vi "SensorIntensidad_Final.vi"() -> ()   [LabVIEW 2024]
uses:
  <vilib>/userDefined/High Color/IMAQdx.ctl
  <vilib>/vision/driver/IMAQdx.llb/IMAQdx Buffer Number Mode.ctl
  <vilib>/vision/driver/IMAQdx.llb/IMAQdx Acquisition Mode.ctl
  <vilib>/express/express shared/transition.llb/Dynamic To Waveform Array.vi
  <vilib>/express/express signal manip/GetorSetDDTAttributes/Set DDT Attributes/SetT0.vi
  <vilib>/express/express shared/transition.llb/Waveform Array To Dynamic.vi
  <vilib>/express/express signal manip/GetorSetDDTAttributes/Set DDT Attributes/Set DDT Properties.xnode
  <vilib>/vision/driver/NI_Vision_Acquisition_Software.lvlib
  <vilib>/vision/NI_Vision_Development_Module.lvlib
panel:
  out "XY Graph":cluster{"Run Time (ms)":u32, "IM":sgl}[](graph)
  out "IM":sgl
  out "Rec":T1 {"Rotation" format="%.2f"; "Left" scale=0.0..1024.0; "Right" scale=0.0..1024.0}
  in  "Buffer Mode":T2
  in  "Cancel Button":bool
  out "frame rate (fps)":u32
  out "Run Time (ms)":u32
  out "ms timer":u32
  in  "Session In":T3
  out "Image":T4(plugin-control)
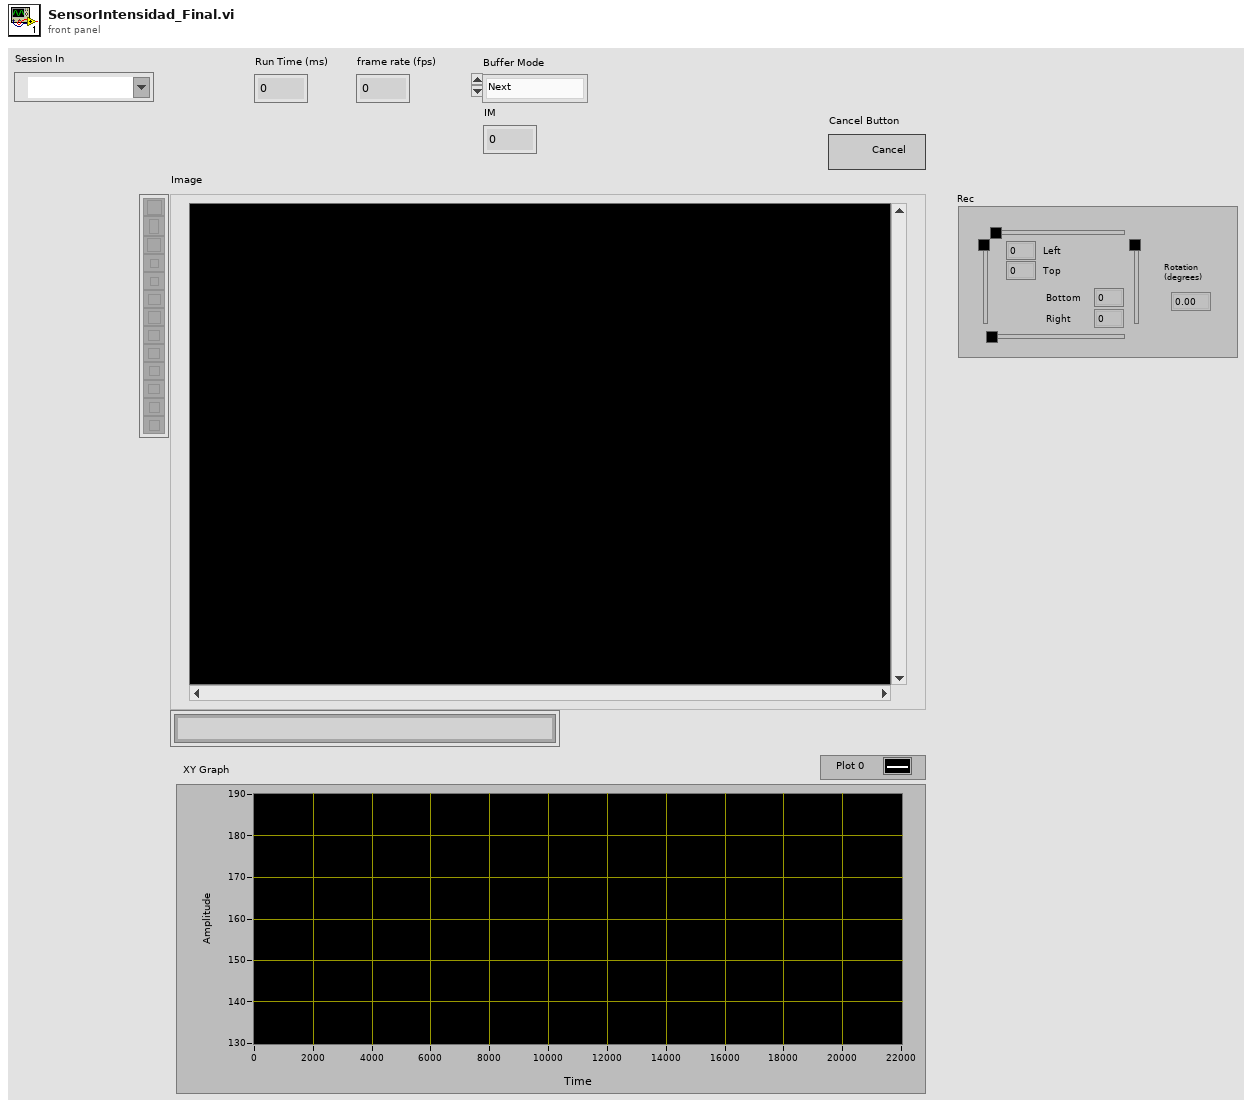
[diagram p1: front panel]
types:
  T1 = typedef "IMAQ Rectangle" = cluster{"Left":i32, "Top":i32, "Right":i32, "Bottom":i32, "Rotation":dbl}
  T2 = typedef "NI_Vision_Acquisition_Software.lvlib/IMAQdx Buffer Number Mode.ctl" = enum32{"Next", "Last", "Buffer Number", "Every", "Last New"}
  T3 = typedef "IMAQdx.ctl" = refnum<k21>
  T4 = typedef "IMAQ Image.ctl" = refnum<image>
  T5 = typedef "Image Type" = u32
  T6 = typedef "NI_Vision_Acquisition_Software.lvlib/IMAQdx Acquisition Mode.ctl" = enum32{"One Shot", "Continuous"}
  T7 = cluster{"Global Rectangle":i32[], "Contours":cluster{"Contour Type":u32, "ROI Type":u32, "Points":i32[]}[]}
  T8 = cluster{"Mean Intensity":sgl, "Standard  Deviation":sgl, "Minimum Intensity":sgl, "Maximum Intensity":sgl}
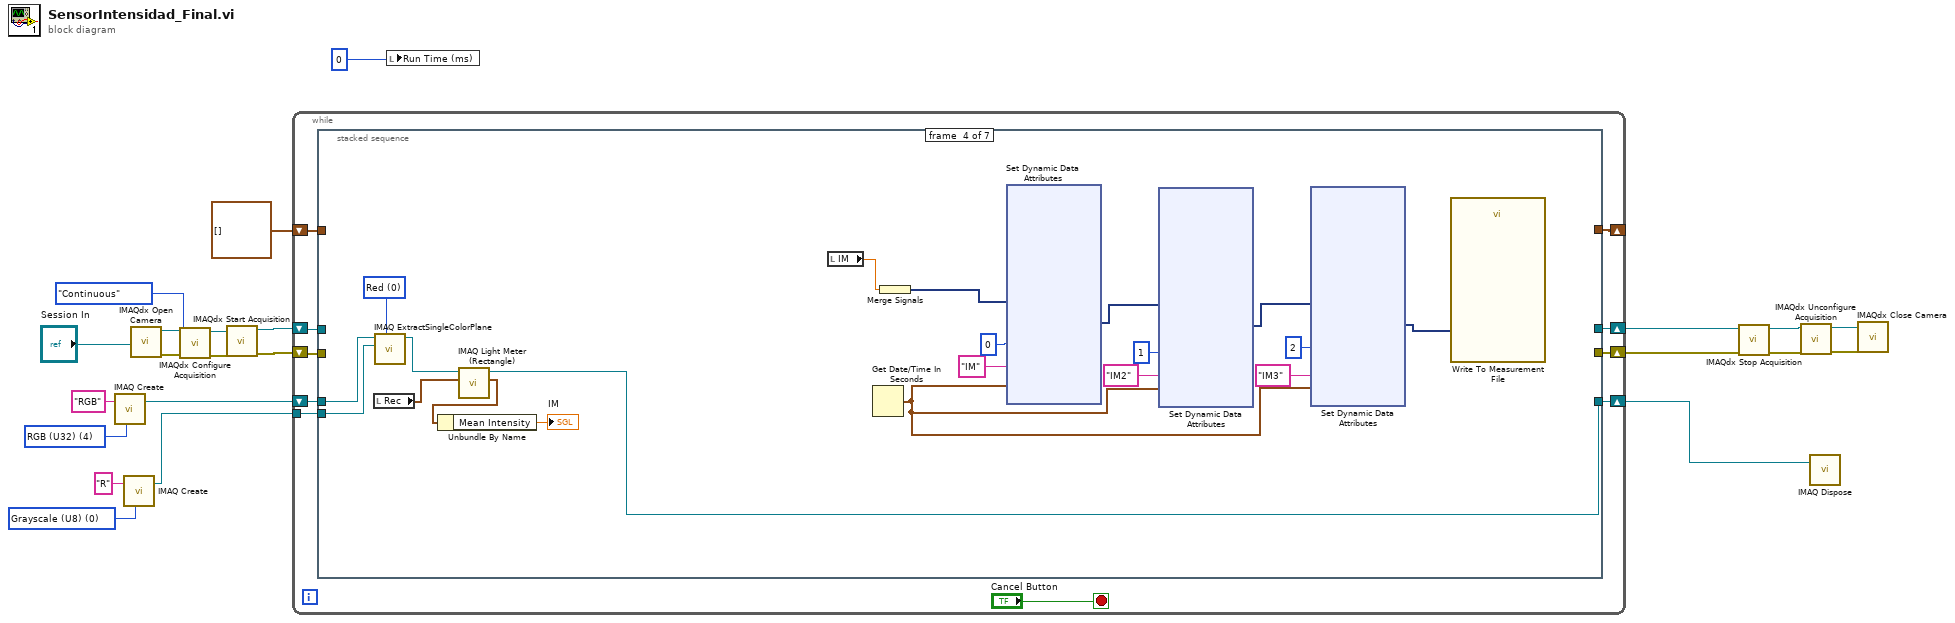
[diagram p0: block diagram]
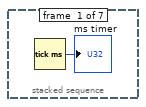
[diagram p2: hidden frame]
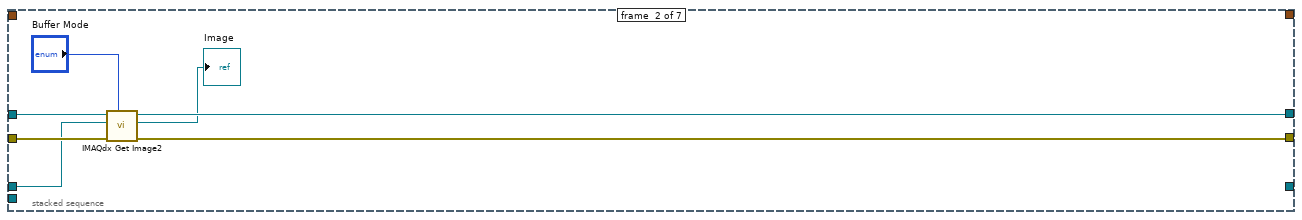
[diagram p3: hidden frame]
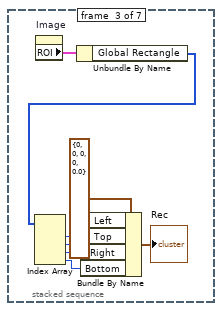
[diagram p4: hidden frame]
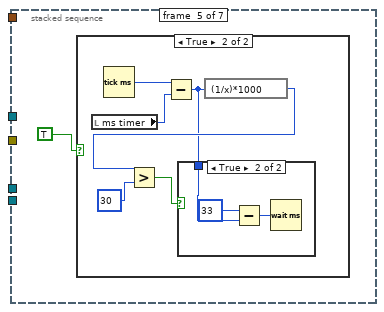
[diagram p5: hidden frame]
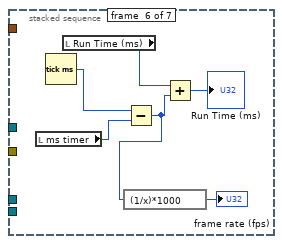
[diagram p8: hidden frame]
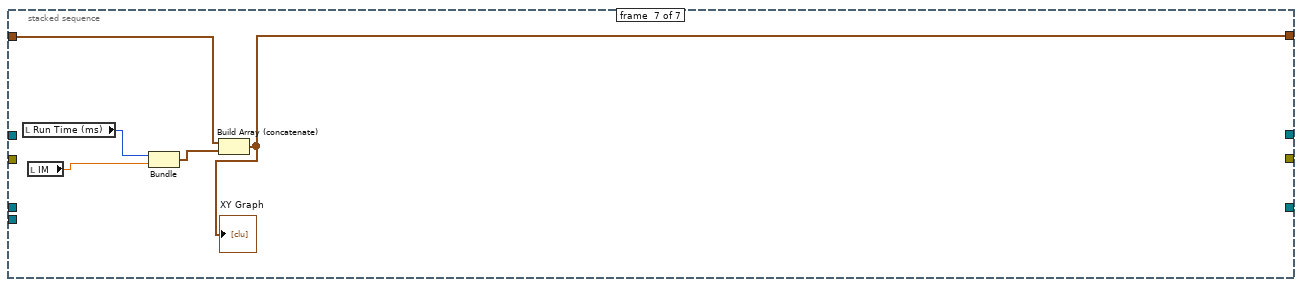
[diagram p9: hidden frame]
diagram:
  w2 = T5 0 items=["Grayscale (U8)", "Grayscale (I16)", "Grayscale (SGL)", "Complex (CSG)", "RGB (U32)", "HSL (U32)", "RGB (U64)", "Grayscale (U16)"] ("Image Type")
  w12 = T5 4 items=["Grayscale (U8)", "Grayscale (I16)", "Grayscale (SGL)", "Complex (CSG)", "RGB (U32)", "HSL (U32)", "RGB (U64)", "Grayscale (U16)"] ("Image Type")
  n1 = call "IMAQ Create"("Image Name"="RGB", "Image Type"=w12) -> ("New Image"=w11:T4)  [unwired: 3 in, 1 out]
  n2 = call "IMAQ Create"("Image Name"="R", "Image Type"=w2) -> ("New Image"=w1:T4)  [unwired: 3 in, 1 out]
  n3 = call <vilib>:"IMAQdx Open Camera.vi"("Session In"="Session In") -> ("error out"=w22:errorcluster, "Session Out"=w23:T3)  [unwired: 9 in]
  n4 = call <vilib>:"IMAQdx Configure Acquisition.vi"("error in"=w22, "Continuous?"=IMAQdx_Acquisition_Mode."Continuous", "Session In"=w23) -> ("error out"=w20:errorcluster, "Session Out"=w21:T3)  [unwired: 7 in]
  n5 = call <vilib>:"IMAQdx Start Acquisition.vi"("error in"=w20, "Session In"=w21) -> ("error out"=w18:errorcluster, "Session Out"=w19:T3)  [unwired: 8 in]
  n6 = while {
    shift-right: [w30] -> w10
    shift-left: w19 -> [w33]
    shift-right: [w29] -> w9
    shift-left: w18 -> [w32]
    shift-right: [w27] -> _
    shift-left: cluster{"Run Time (ms)":u32, "IM":sgl}[] [] -> [w26]
    shift-right: [w25] -> w4
    shift-left: w11 -> [w31]
    tunnel: w1 -> [w24]
    stop <- "Cancel Button" stop-if-true
    n7 = stacked-sequence {
      tunnel: w33 -> [_ w41 _ _ _ _ _]
      tunnel: w32 -> [_ w40 _ _ _ _ _]
      tunnel: w31 -> [_ w39 _ w66 _ _ _]
      tunnel: [_ w38 _ _ _ _ _] -> w30
      tunnel: [_ w37 _ _ _ _ _] -> w29
      tunnel: [_ _ _ _ _ _ w139] -> w27
      tunnel: w26 -> [_ _ _ _ _ _ w138]
      tunnel: [_ _ _ w65 _ _ _] -> w25
      tunnel: w24 -> [_ _ _ w63 _ _ _]
      frame #0 {
        n8 = Tick Count (ms)() -> (millisecond timer value=→"ms timer":u32)
      }
      frame #1 {
        n9 = call <vilib>:"IMAQdx Get Image2.vi"("Buffer Number Mode (Next)"="Buffer Mode", "error in"=w40, "Image In"=w39, "Session In"=w41) -> ("error out"=w37:errorcluster, "Image Out"=→"Image":T4, "Session Out"=w38:T3)  [unwired: 4 in, 1 out]
      }
      frame #2 {
        n10 = property on="Image" class="ImageControl"() -> ("ROI"=w49:T7)  [unwired: 2 in, 2 out]
        n11 = Unbundle By Name(w49) -> ("Global Rectangle"=w42:i32[])
        n12 = Index Array(array=w42) -> (element #1=w47:i32, element #2=w46:i32, element #3=w45:i32, element #4=w44:i32)  [unwired: 4 in]
        n13 = Bundle By Name(cluster=T1 {"Left"=0, "Top"=0, "Right"=0, "Bottom"=0, "Rotation"=0.0} ("Rectangle"), "Left"=w47, "Top"=w46, "Right"=w45, "Bottom"=w44) -> (→"Rec":T1)
      }
      frame #3 {
        w64 = 0 items=["Red", "Green", "Blue", "Hue", "Saturation", "Luminance", "Value", "Intensity"] ("Color Plane")
        n14 = local read "Rec"() -> (w69:T1)
        n15 = call "IMAQ ExtractSingleColorPlane"("Color Plane"=w64, "Image Dst"=w63, "Image Src"=w66) -> ("Image Dst Out"=w58:T4)  [unwired: 7 in, 1 out]
        n16 = call "IMAQ Light Meter (Rectangle)"("Rectangle"=w69, "Image"=w58) -> ("Gray Level Intensities"=w68:T8, "Image Out"=w65:T4)  [unwired: 5 in, 3 out]
        n17 = Unbundle By Name(w68) -> ("Mean Intensity"=→"IM":sgl)
        n18 = local read "IM"() -> (w59:sgl)
        n19 = Get Date/Time In Seconds() -> (seconds since 1Jan1904=w55:timestamp)
        n20 = Merge Signals(w59) -> (w62:dynamicdata)
        n21 = xnode "Set Dynamic Data Attributes"("Signals In"=w62, "Signal Index"=0, "Signal Name"="IM", "Timestamp"=w55) -> ("Signals Out"=w52:dynamicdata)  [unwired: 1 in, 1 out]
        n22 = xnode "Set Dynamic Data Attributes"("Signals In"=w52, "Signal Index"=1, "Signal Name"="IM2", "Timestamp"=w55) -> ("Signals Out"=w51:dynamicdata)  [unwired: 1 in, 1 out]
        n23 = xnode "Set Dynamic Data Attributes"("Signals In"=w51, "Signal Index"=2, "Signal Name"="IM3", "Timestamp"=w55) -> ("Signals Out"=w50:dynamicdata)  [unwired: 1 in, 1 out]
        n24 = call "Write To Measurement File"("Signals"=w50) -> ()  [unwired: 16 in, 3 out]
      }
      frame #4 {
        n25 = case shown="True" TRUE {
          frame False {
          }
          frame True {
            n26 = local read "ms timer"() -> (w126:u32)
            n27 = Tick Count (ms)() -> (millisecond timer value=w127:u32)
            n28 = Subtract(x=w127, y=w126) -> (x-y=w123:u32)
            n29 = expression code="(1/x)*1000"(w123) -> (w125:u32)
            n30 = Greater?(x=w125, y=u32 30) -> (0:w122:bool)
            n31 = case shown="True" w122 {
              tunnel: w123 -> [_ w130]
              frame False {
              }
              frame True {
                n32 = Subtract(x=u32 33, y=w130) -> (x-y=w128:u32)
                n33 = Wait (ms)(milliseconds to wait=w128) -> ()  [unwired: 1 out]
              }
            }
          }
        }
      }
      frame #5 {
        n34 = local read "ms timer"() -> (w136:u32)
        n35 = Tick Count (ms)() -> (millisecond timer value=w135:u32)
        n36 = local read "Run Time (ms)"() -> (w133:u32)
        n37 = Subtract(x=w135, y=w136) -> (x-y=w132:u32)
        n38 = expression code="(1/x)*1000"(w132) -> (→"frame rate (fps)":u32)
        n39 = Add(x=w133, y=w132) -> (x+y=→"Run Time (ms)":u32)
      }
      frame #6 {
        n40 = local read "Run Time (ms)"() -> (w141:u32)
        n41 = local read "IM"() -> (w137:sgl)
        n42 = Bundle("Run Time (ms)"=w141, "IM"=w137) -> (w140:cluster{"Run Time (ms)":u32, "IM":sgl})  [unwired: 1 in]
        n43 = Build Array (concatenate)(w138, w140) -> (w139:cluster{"Run Time (ms)":u32, "IM":sgl}[])
        "XY Graph" <- w139
      }
    }
  }
  n44 = local write "Run Time (ms)"(u32 0 ("Run Time")) -> ()
  n45 = call <vilib>:"IMAQdx Stop Acquisition.vi"("error in"=w9, "Session In"=w10) -> ("error out"=w16:errorcluster, "Session Out"=w17:T3)  [unwired: 8 in]
  n46 = call <vilib>:"IMAQdx Unconfigure Acquisition.vi"("error in"=w16, "Session In"=w17) -> ("error out"=w15:errorcluster, "Session Out"=w14:T3)  [unwired: 8 in]
  n47 = call "IMAQ Dispose"("Image"=w4) -> ()  [unwired: 5 in, 1 out]
  n48 = call <vilib>:"IMAQdx Close Camera.vi"("error in"=w15, "Session In"=w14) -> ()  [unwired: 9 in, 1 out]
